vi "Get Stream.vi"(8 "error in (no error)":errorcluster, 11 "TCP Client in":refnum<class "TCP Client.lvclass">) -> (0 "error out":errorcluster, 2 "Stream":refnum<class "Stream.lvclass">, 3 "TCP Client out":refnum<class "TCP Client.lvclass">)   [LabVIEW 2020, in "Stream-TCP.lvlib" / "TCP Client.lvclass"]
uses:
  TCP Client.lvclass
  lv-stream/stream/Stream/Stream.lvclass
  TCP Client.lvclass/TCP Client.ctl
  TCP Stream/TCP Stream.lvclass
  C:/dev/LabVIEW/lv-stream/stream/Stream/Stream.lvclass
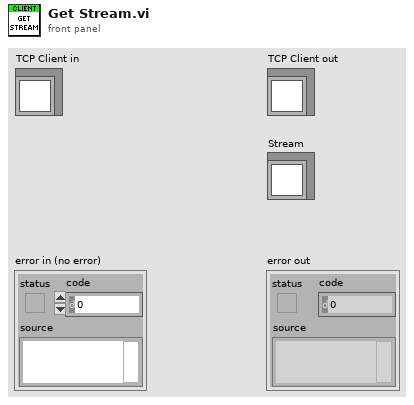
[diagram p1: front panel]
types:
  T1 = typedef "Stream-TCP.lvlib/TCP Client.lvclass/Ref Data.ctl" = cluster{"TCP Connection":refnum<k5>, "TCP Stream":refnum<class "TCP Stream.lvclass">, "State":T2, "Connection Loop":refnum<vi>, "TCP Mode":T3, "Timeout ms":i32, "Server Connection":bool}
  T2 = typedef "Stream-TCP.lvlib/TCP Client.lvclass/Connection State.ctl" = enum16{"Closed", "Idle", "Connecting", "Connected", "Shutdown"}
  T3 = typedef "Stream-TCP.lvlib/TCP Mode.ctl" = enum16{"buffered", "raw"}
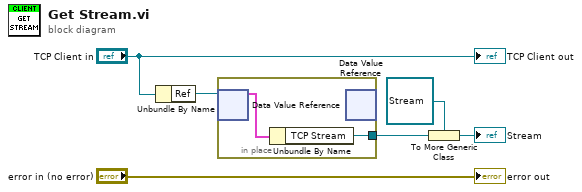
[diagram p0: block diagram]
diagram:
  n1 = Unbundle By Name("TCP Client in") -> ("Ref"=w6:refnum<data-value>)
  n2 = in-place {
    in-place-border: [w7] -> w4
    n3 = in-place-dvr #1(w6) -> (w8:T1)  [unwired: 1 out]
    n4 = Unbundle By Name(w8) -> ("TCP Stream"=w7:refnum<class "TCP Stream.lvclass">)
    n5 = in-place-dvr #1() -> ()  [unwired: 1 in, 2 out]
  }
  n6 = To More Generic Class(target class=refnum<class "Stream.lvclass"> refnum ("Stream.lvlib:Stream.lvclass"), reference=w4) -> (generic class reference=→"Stream":refnum<class "Stream.lvclass">)
  "error out" <- "error in (no error)"
  "TCP Client out" <- "TCP Client in"
